vi "VNA.Write Configuration.vi"(8 "error in (no error)":errorcluster, 10 "Configuration":T1, 11 "VNA":refnum<class "VNA.lvclass">) -> (0 "error out":errorcluster, 3 "VNA out":refnum<class "VNA.lvclass">)   [LabVIEW 2016, in "VNA.lvclass"]
uses:
  VNA.lvclass
  Typedefs/VNA.Configuration--Cluster.ctl
  VNA.lvclass/VNA.ctl
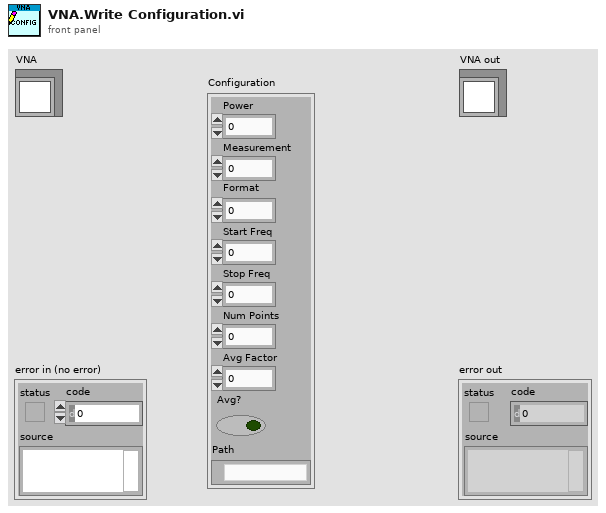
[diagram p1: front panel]
types:
  T1 = typedef "VNA.lvclass/VNA.Configuration--Cluster.ctl" = cluster{"Power":dbl, "Measurement":dbl, "Format":dbl, "Start Freq":dbl, "Stop Freq":dbl, "Num Points":dbl, "Avg Factor":dbl, "Avg?":bool, "Path":path}
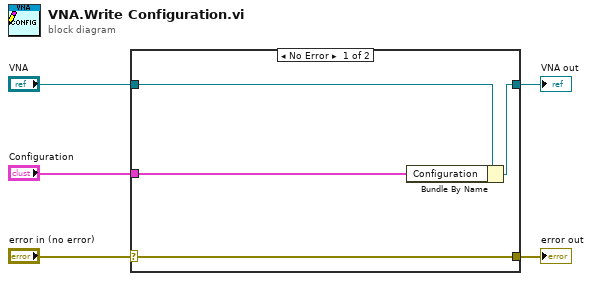
[diagram p0: block diagram]
diagram:
  n1 = case shown="No Error" "error in (no error)" {
    selector: "error in (no error)" -> [w9 w10]
    tunnel: [w9 w10] -> w4
    tunnel: [w7 w11] -> w2
    tunnel: "VNA" -> [w8 w11]
    tunnel: "Configuration" -> [w6 _]
    frame No Error {
      n2 = Bundle By Name(cluster=w8, "Configuration"=w6) -> (w7:refnum<class "VNA.lvclass">)
    }
    frame Error {
    }
  }
  "error out" <- w4
  "VNA out" <- w2
